vi "GuardarColores.vi"   [LabVIEW 2017]
uses:
  Control/Enum_GuardarColores.ctl
types:
  T1 = typedef "Enum_GuardarColores.ctl" = enum16{"Default", "Stop", "Mostrar", "Guardar", "Reiniciar"}
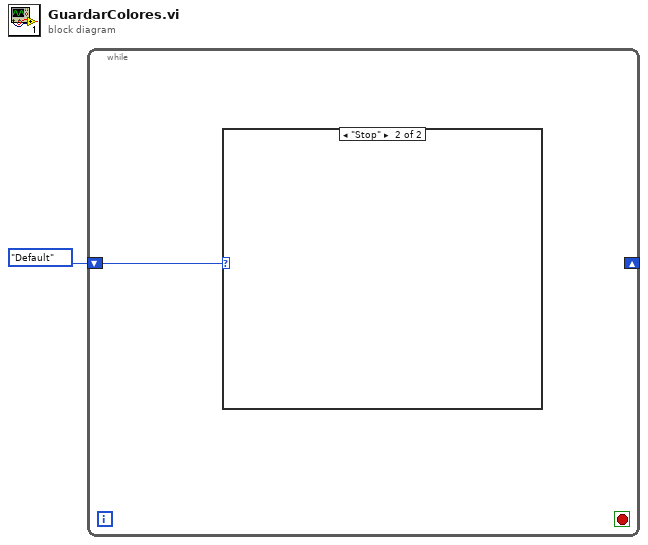
[diagram p0: block diagram]
diagram:
  n1 = while {
    shift-right: _ -> [_]
    shift-left: Enum_GuardarColores."Default" -> [w2]
    stop <- _ stop-if-true
    n2 = case shown="\"Stop\"" w2 {
      frame "Default", Default {
      }
      frame "Stop" {
      }
    }
  }
